vi "QTrkSetZLUT.vi"(6 "Normalize LUT":bool, 8 "error in (no error)":errorcluster, 9 "Z Compare window (default: stetson)":sgl[](array[numeric]), 10 "ZLUT":sgl[][][](array[numeric]), 11 "QTrk Instance":T1) -> (0 "error out":errorcluster, 3 "QTrk Instance":T1)   [LabVIEW 2011]
uses:
  QTrkInstance.ctl
  QTrkDLL.vi
panel:
  out "zcmpWindow":sgl[](array[numeric])
  out "Waveform Graph":sgl[](graph)
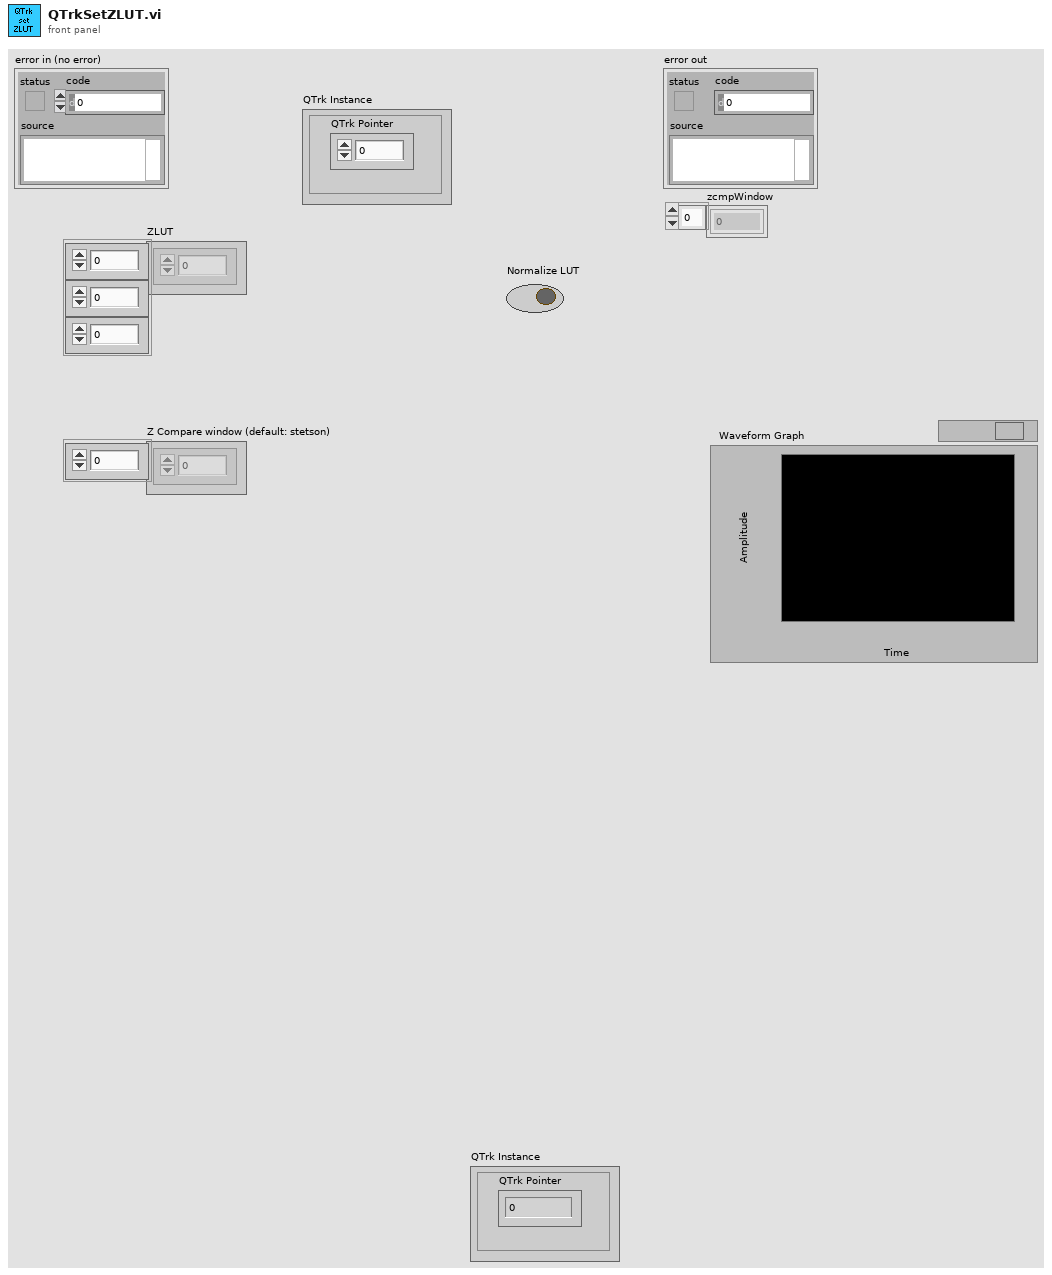
[diagram p1: front panel]
types:
  T1 = typedef "QTrkInstance.ctl" = cluster{"QTrk Pointer":u64}
  T2 = typedef "QTrkComputedSettings.ctl" = cluster{"QTrk Settings":T3, "Derived settings":cluster{"ZLUT Radial Steps":i32, "ZLUT Angular Steps":i32, "ZLUT Max Radius":sgl, "QI Radial Steps":i32, "QI Angular Steps\nPer Quadrant":i32, "QI Max Radius":sgl}}
  T3 = typedef "QTrkSettings.ctl" = cluster{"Image width":i32, "Image height":i32, "Number of threads (CPU based)":i32, "CUDA Device":i32, "COM Background correction factor":sgl, "ZLUT MinRadius":sgl, "ZLUT Radial sample density":sgl, "ZLUT Angular sample density":sgl, "ZLUT ROI Coverage":sgl, "QI Iterations":i32, "QI MinRadius":sgl, "QI Radial sample density":sgl, "QI Angular sample density":sgl, "QI ROI Coverage":sgl, "QI Angular Step \nIteration Factor":sgl, "XCOR Profile Length":i32, "XCOR Profile Width":i32, "XCOR Iterations":i32, "Gaussian 2D Fit Iterations":i32, "Gaussian 2D Sigma (pixels)":sgl, "Downsample":i32}
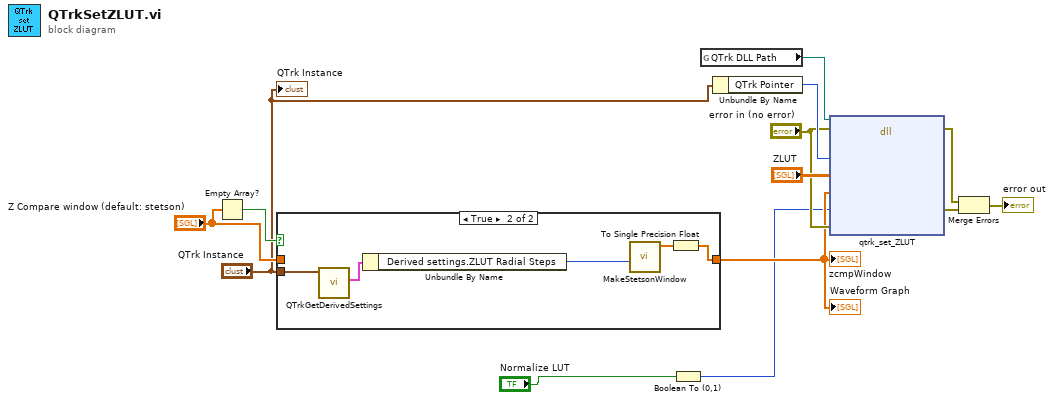
[diagram p0: block diagram]
diagram:
  n1 = Empty Array?(array="Z Compare window (default: stetson)") -> (empty?=w5:bool)
  n2 = case shown="True" w5 {
    tunnel: [w14 w17] -> w4
    tunnel: "Z Compare window (default: stetson)" -> [w14 _]
    tunnel: "QTrk Instance" -> [_ w16]
    frame False {
    }
    frame True {
      n3 = call "QTrkGetDerivedSettings.vi"("QTrk Instance"=w16) -> ("Derived settings"=w15:T2)  [unwired: 5 in, 5 out]
      n4 = Unbundle By Name(w15) -> ("Derived settings.ZLUT Radial Steps"=w19:i32)
      n5 = call "MakeStetsonWindow.vi"("radialsteps"=w19) -> ("Window"=w18:dbl[])  [unwired: 10 in]
      n6 = To Single Precision Float(number=w18) -> (single precision float=w17:sgl[])
    }
  }
  "Waveform Graph" <- w4
  "zcmpWindow" <- w4
  n7 = Boolean To (0,1)(Boolean="Normalize LUT") -> (0, 1=w1:i16)
  n8 = global read "QTrkDLL.vi" "QTrk DLL Path"() -> (w11:path)
  n9 = Unbundle By Name("QTrk Instance") -> ("QTrk Pointer"=w13:u64)
  n10 = dll-call lib="D:/jcnossen1/cudaqi-tracker/bin/jtrk-labview.dll" fn="qtrk_set_ZLUT"(path in=w11, error in="error in (no error)", "tracker"=w13, "zlut"="ZLUT", "zcmpWindow"=w4, "renormalize"=w1, "error"="error in (no error)") -> (error out=w9:errorcluster, "error"=w8:errorcluster)  [unwired: 6 in, 1 out]
  n11 = Merge Errors(w9, w8) -> (→"error out":errorcluster)
  "QTrk Instance" <- "QTrk Instance"
